vi "INI Loader.vi"(8 "error in (no error)":errorcluster, 11 "Father Of All Detectors in":refnum<class "Father Of All Detectors.lvclass">) -> (0 "error out":errorcluster, 3 "Father Of All Detectors out":refnum<class "Father Of All Detectors.lvclass">)   [LabVIEW 2026, in "TALOS.lvlib" / "Father Of All Detectors.lvlib" / "Father Of All Detectors.lvclass"]
uses:
  Father Of All Detectors.lvclass
  Father Of All Detectors.lvclass/Father Of All Detectors.ctl
  Config/Config.lvclass
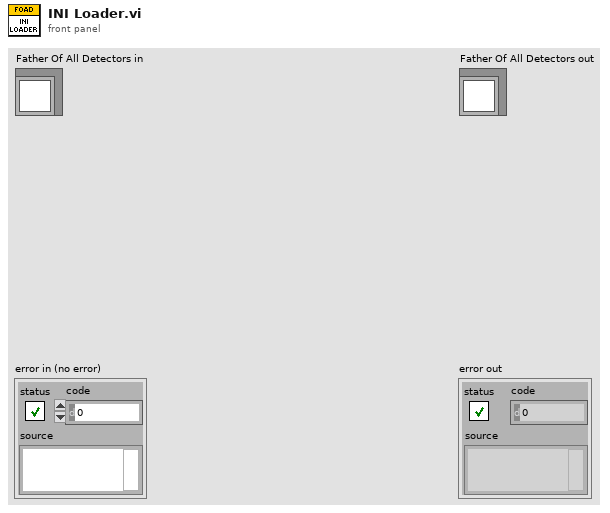
[diagram p1: front panel]
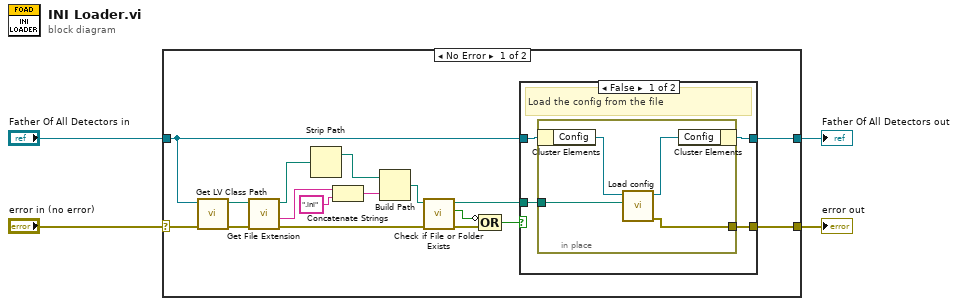
[diagram p0: block diagram]
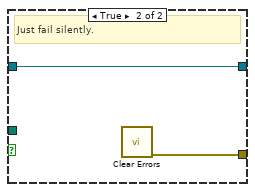
[diagram p2: hidden frame]
diagram:
  n1 = case shown="No Error" "error in (no error)" {
    selector: "error in (no error)" -> [w21 w33]
    tunnel: [w16 w33] -> w3
    tunnel: [w17 w32] -> w1
    tunnel: "Father Of All Detectors in" -> [w18 w32]
    frame No Error {
      n2 = call <vilib>:"Get LV Class Path.vi"("error in (no error)"=w21, "object"=w18) -> ("error out"=w20:errorcluster, "class path"=w19:path)  [unwired: 8 in]
      n3 = call <vilib>:"Get File Extension.vi"("error in (no error)"=w20, "file"=w19) -> ("error out"=w10:errorcluster, "filename without extension"=w13:string, "dup file"=w11:path)  [unwired: 5 in, 2 out]
      n4 = Strip Path(path=w11) -> (stripped path=w15:path)  [unwired: 1 out]
      n5 = Concatenate Strings(w13, ".ini" ("string")) -> (w14:string)
      n6 = Build Path(base path=w15, name or relative path=w14) -> (appended path=w9:path)
      n7 = call <vilib>:"Check if File or Folder Exists.vi"("error in (no error)"=w10, "path"=w9) -> ("error out"=w7:errorcluster, "file or folder exists?"=w6:bool, "dup path"=w8:path)  [unwired: 7 in]
      n8 = Compound Arithmetic op=OR(invert w6, w7) -> (w5:bool)
      n9 = case shown="False" w5 {
        tunnel: w18 -> [w25 w31]
        tunnel: [w23 w31] -> w17
        tunnel: [w24 w30] -> w16
        tunnel: w8 -> [w22 _]
        frame False {
          # "Load the config from the file"
          n10 = in-place {
            in-place-border: [w27] -> w24
            in-place-border: w22 -> [w26]
            n11 = in-place-cluster #1(w25) -> ("Config"=w29:refnum<class "Config.lvclass">)
            n12 = call "Load config.vi"("config file path"=w26, "Config in"=w29) -> ("error out"=w27:errorcluster, "Config out"=w28:refnum<class "Config.lvclass">)  [unwired: 8 in]
            n13 = in-place-cluster #1("Config"=w28) -> (w23:refnum<class "Father Of All Detectors.lvclass">)
          }
        }
        frame True {
          # "Just fail silently."
          n14 = call <vilib>:"Clear Errors.vi"() -> ("error out"=w30:errorcluster)  [unwired: 6 in, 1 out]
        }
      }
    }
    frame Error {
    }
  }
  "error out" <- w3
  "Father Of All Detectors out" <- w1
